vi "Main_RT_Watchdog_Off.vi"() -> ()   [LabVIEW 2015]
uses:
  <vilib>/addons/InsightCM/Devices/Shared/AcquireScanEngine/ScanEngine.lvlib
  <vilib>/addons/InsightCM/Devices/Shared/Trigger/Trigger.lvlib
  <vilib>/addons/InsightCM/Devices/Shared/TdmsCreator/TdmsCreator.lvlib
  <vilib>/addons/TraceLogger/TraceLogger.lvlib
  <vilib>/addons/TimerProcess/TimerProcess.lvlib
  <vilib>/addons/BlinkProcess/BlinkProcess.lvlib
  <vilib>/addons/InsightCM/Devices/Shared/Controller/Controller.lvlib
  <vilib>/addons/InsightCM/Devices/Shared/ServerComm/ServerComm.lvlib
  <vilib>/addons/InsightCM/Devices/Shared/FileManager/FileManager.lvlib
  <vilib>/addons/InsightCM/Devices/Shared/TracePointDisplay/TracePointDisplay.lvlib
  <vilib>/addons/InsightCM/Devices/Shared/TagPublish/TagPublish.lvlib
  <vilib>/addons/InsightCM/Devices/Shared/DataAccumulatorProcess/DataAccumulator.lvlib
  <vilib>/addons/InsightCM/Devices/Shared/DeviceHealth/DeviceHealth.lvlib
  <vilib>/addons/InsightCM/Devices/Shared/SinglePointClock/SinglePointClock.lvlib
  <vilib>/addons/InsightCM/Devices/Shared/VibrationVirtualChannel/VibrationVirtualChannel.lvlib
  <vilib>/addons/InsightCM/Devices/Shared/Alarm/Alarm.lvlib
  <vilib>/addons/InsightCM/Devices/Shared/TestPanel/TestPanel.lvlib
  <vilib>/addons/InsightCM/Devices/Shared/DataExplorerHelper/DataExplorerHelper.lvlib
  <vilib>/addons/InsightCM/Devices/Shared/ModbusMaster/ModbusMaster.lvlib
  <vilib>/addons/WatchdogProcess/WatchdogProcess.lvlib
panel:
  out "debug":string
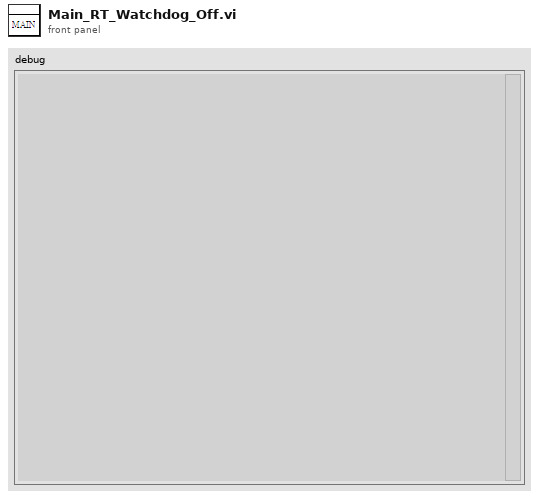
[diagram p1: front panel]
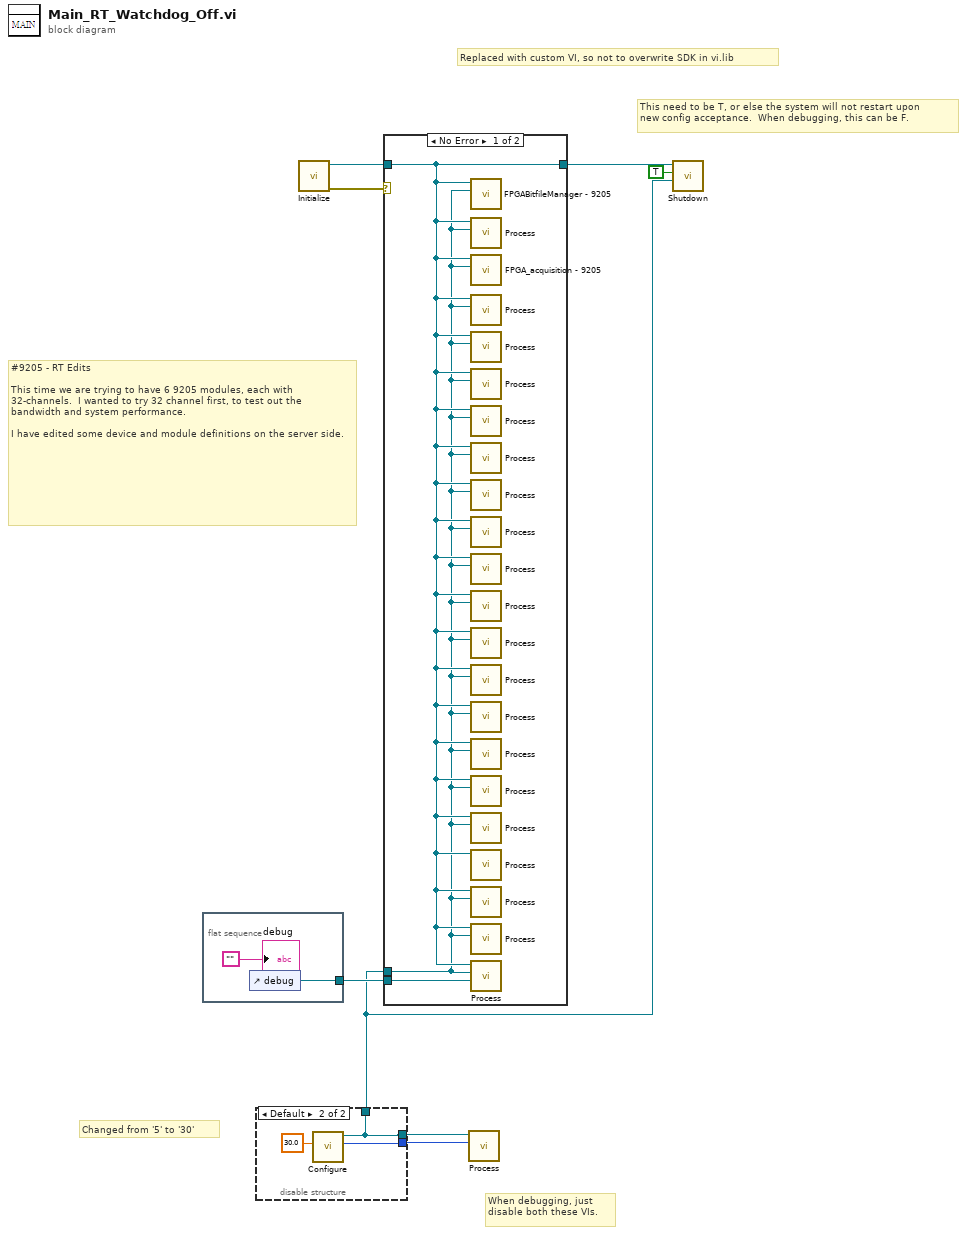
[diagram p0: block diagram]
diagram:
  # "When debugging, just\ndisable both these VIs."
  # "Changed from '5' to '30'"
  # "This need to be T, or else the system will not restart upon\nnew config acceptance.  When debugging, this can be F."
  # "Replaced with custom VI, so not to overwrite SDK in vi.lib"
  # "#9205 - RT Edits\n\nThis time we are trying to have 6 9205 modules, each with 32-channels.  I wanted to try 32 channel first, to test out the bandwidth and system performance.\n  \nI have edited some device and module definitions on the server side."
  n1 = flat-sequence {
    tunnel: [w9] -> w6
    frame #0 {
      n2 = control-ref of="debug"() -> (w9:refnum<vi>)
      "debug" <- ""
    }
  }
  n3 = disable-structure shown="Default" {
    disable-tunnel: [_ w12] -> w4
    disable-tunnel: [_ w12] -> w2
    disable-tunnel: [_ w11] -> w1
    frame condition #0 {
    }
    frame condition #1 (active) {
      n4 = call <vilib>:"Configure.vi"("hw timeout (sec)"=30.0) -> ("watchdogID out"=w11:u64, "Pound"=w12:refnum<class "Pound.lvclass">)  [unwired: 8 in, 1 out]
    }
  }
  n5 = call <vilib>:"Initialize.vi"() -> ("error out"=w8:errorcluster, "Qbus out"=w5:refnum<class "Qbus.lvclass">)  [unwired: 10 in]
  n6 = case shown="No Error" w8 {
    tunnel: w5 -> [w15 w17]
    tunnel: [w15 w17] -> w7
    tunnel: w4 -> [w14 _]
    tunnel: w6 -> [w16 _]
    frame No Error {
      n7 = call "FPGABitfileManager - 9205.vi"("Pound in"=w14, "Qbus in"=w15) -> ()  [unwired: 9 in, 1 out]
      n8 = call <vilib>:"Process.vi"("Pound in"=w14, "Qbus in"=w15) -> ()  [unwired: 9 in, 1 out]
      n9 = call "FPGA_acquisition - 9205.vi"("pound in"=w14, "qbus in"=w15) -> ()  [unwired: 9 in, 1 out]
      n10 = call <vilib>:"Process.vi"("Pound in"=w14, "Qbus in"=w15) -> ()  [unwired: 9 in, 1 out]
      n11 = call <vilib>:"Process.vi"("pound in"=w14, "qbus in"=w15) -> ()  [unwired: 9 in, 1 out]
      n12 = call <vilib>:"Process.vi"("Pound in"=w14, "Qbus in"=w15) -> ()  [unwired: 9 in, 1 out]
      n13 = call <vilib>:"Process.vi"("pound in"=w14, "Qbus in"=w15) -> ()  [unwired: 9 in, 1 out]
      n14 = call <vilib>:"Process.vi"("Pound in"=w14, "Qbus in"=w15) -> ()  [unwired: 9 in, 1 out]
      n15 = call <vilib>:"Process.vi"("Pound in"=w14, "Qbus in"=w15) -> ()  [unwired: 9 in, 1 out]
      n16 = call <vilib>:"Process.vi"("Pound in"=w14, "Qbus in"=w15) -> ()  [unwired: 9 in, 1 out]
      n17 = call <vilib>:"Process.vi"("Pound in"=w14, "Qbus in"=w15) -> ()  [unwired: 9 in, 1 out]
      n18 = call <vilib>:"Process.vi"("Pound in"=w14, "Qbus in"=w15) -> ()  [unwired: 9 in, 1 out]
      n19 = call <vilib>:"Process.vi"("Pound in"=w14, "Qbus in"=w15) -> ()  [unwired: 9 in, 1 out]
      n20 = call <vilib>:"Process.vi"("Pound in"=w14, "Qbus in"=w15) -> ()  [unwired: 9 in, 1 out]
      n21 = call <vilib>:"Process.vi"("Pound in"=w14, "Qbus in"=w15) -> ()  [unwired: 9 in, 1 out]
      n22 = call <vilib>:"Process.vi"("Pound in"=w14, "Qbus in"=w15) -> ()  [unwired: 9 in, 1 out]
      n23 = call <vilib>:"Process.vi"("Pound in"=w14, "Qbus in"=w15) -> ()  [unwired: 9 in, 1 out]
      n24 = call <vilib>:"Process.vi"("Pound in"=w14, "Qbus in"=w15) -> ()  [unwired: 9 in, 1 out]
      n25 = call <vilib>:"Process.vi"("qbus in"=w15) -> ()  [unwired: 10 in, 1 out]
      n26 = call <vilib>:"Process.vi"("Pound"=w14, "Qbus in"=w15) -> ()  [unwired: 9 in, 1 out]
      n27 = call <vilib>:"Process.vi"("pound in"=w14, "qbus in"=w15) -> ()  [unwired: 9 in, 1 out]
      n28 = call <vilib>:"Process.vi"("string refnum"=w16, "Pound in"=w14, "Qbus in"=w15) -> ()  [unwired: 8 in, 1 out]
    }
    frame Error {
    }
  }
  n29 = call <vilib>:"Process.vi"("watchdogID"=w1, "Pound"=w2) -> ()  [unwired: 7 in, 3 out]
  n30 = call <vilib>:"Shutdown.vi"("Pound"=w4, "restart system"=TRUE, "Qbus in"=w7) -> ()  [unwired: 8 in, 1 out]
